vi "TerminateErrorProcessor.vi"(7 "priority (-1, highest)":i32=-1, 8 "error in":errorcluster, 11 "error processor in":refnum<class "ErrorProcessor.lvclass">) -> (0 "error out":errorcluster, 2 "message sent?":bool)   [LabVIEW 2013, in "CLM_ErrorHandler.lvlib" / "ErrorProcessor.lvclass"]
uses:
  ErrorProcessor.lvclass
  ErrorProcessor.lvclass/ErrorProcessor.ctl
  ErrorReporter/ErrorReporter.lvclass
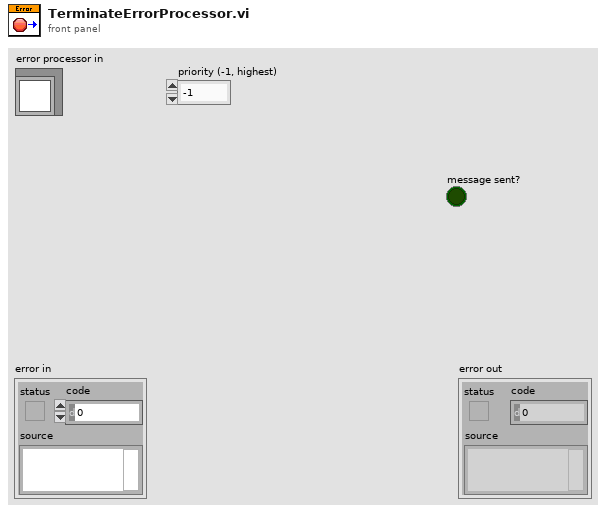
[diagram p1: front panel]
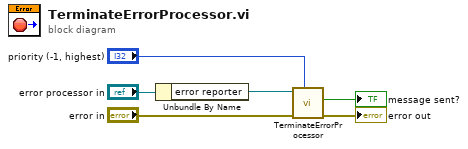
[diagram p0: block diagram]
diagram:
  n1 = Unbundle By Name("error processor in") -> ("error reporter"=w5:refnum<class "ErrorReporter.lvclass">)
  n2 = call "TerminateErrorProcessor.vi"("priority (-1, highest)"="priority (-1, highest)", "error in"="error in", "error reporter in"=w5) -> ("error out"=→"error out":errorcluster, "message sent?"=→"message sent?":bool)  [unwired: 7 in]
